vi "Puff_using_Arduino_oneshot.vi"(0 "Puff_duration:Sec":dbl=1.0 format="%.2g") -> ()   [LabVIEW 2015]
uses:
  Controls/Post_Process.ctl
  Controls/Setup.ctl
  Globals/Meas_global.vi
panel:
  out "Puff Time used":dbl=1.0 format="%.2g"
  out "Case Currently On":string="Loop"
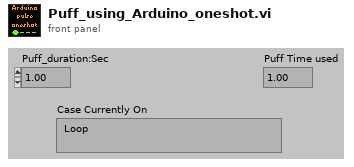
[diagram p1: front panel]
types:
  T1 = typedef "Setup.ctl" = enum16{"Run Program", "Show Setup", "Save Current Setup", "Setup Front Panel"}
  T2 = typedef "Post_Process.ctl" = enum16{"Take New Data", "Post Process Raw Data File"}
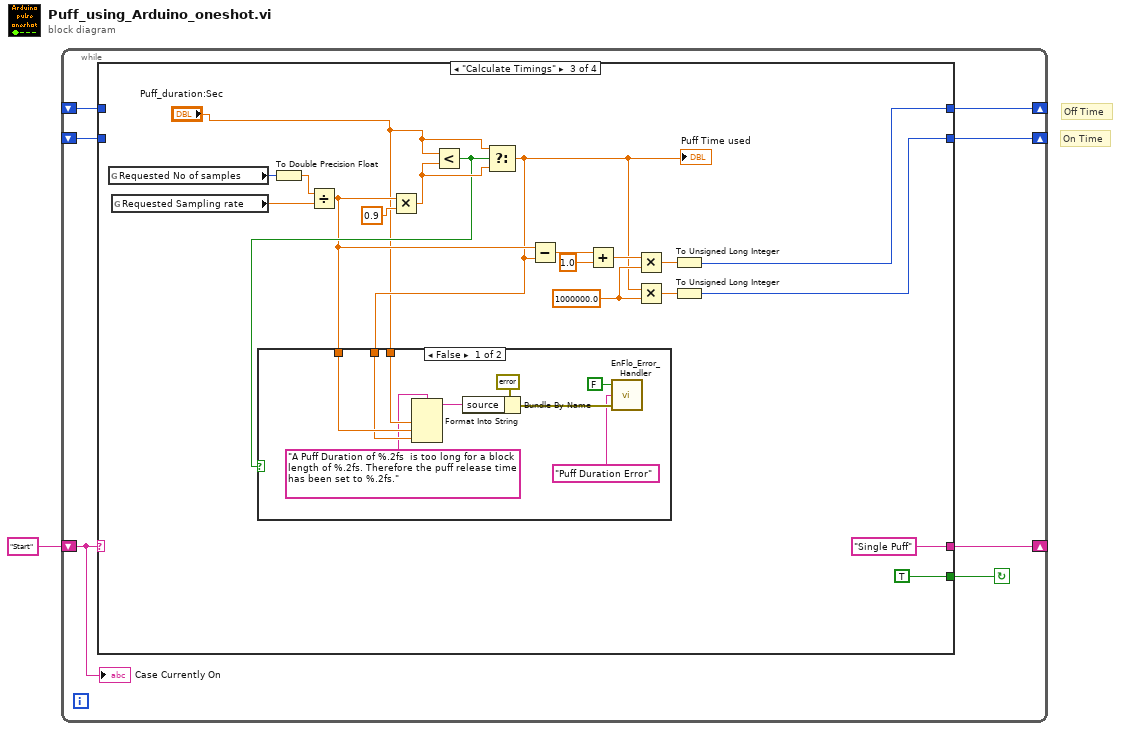
[diagram p0: block diagram]
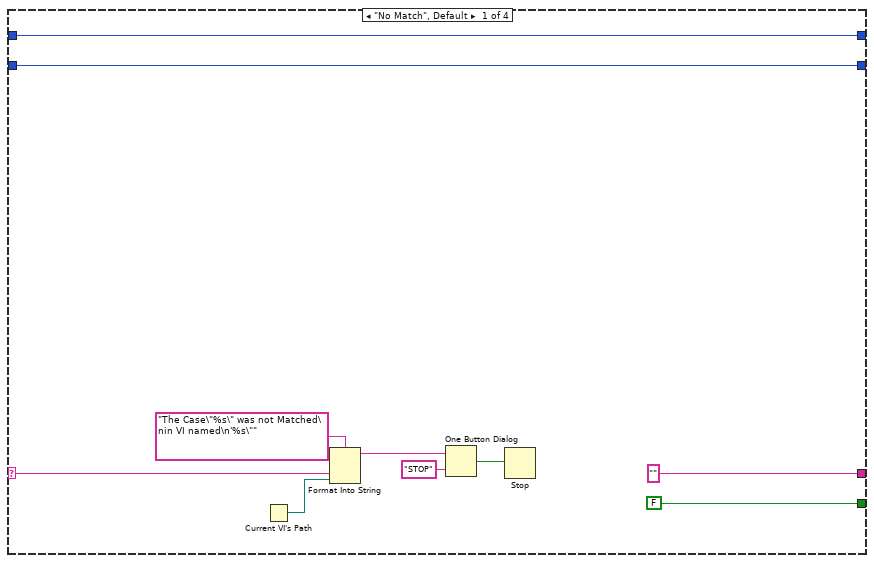
[diagram p2: hidden frame]
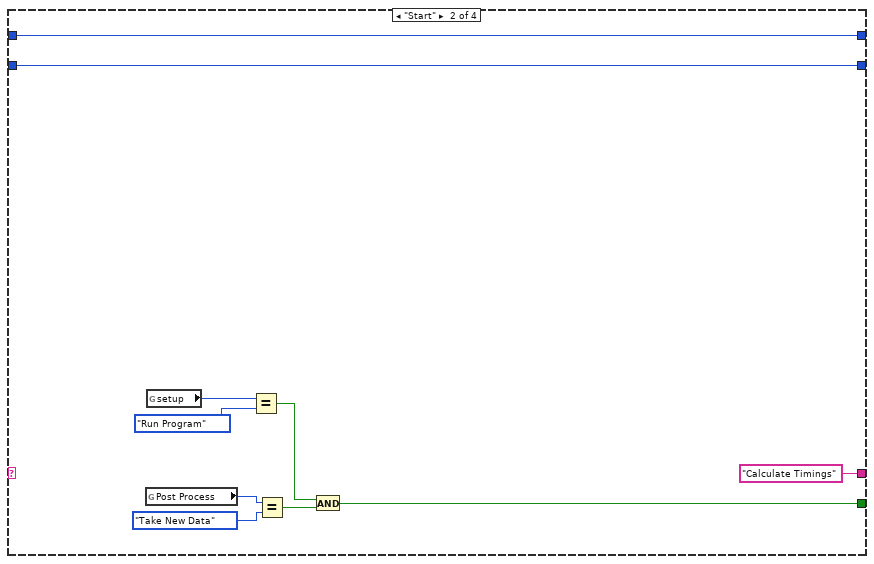
[diagram p3: hidden frame]
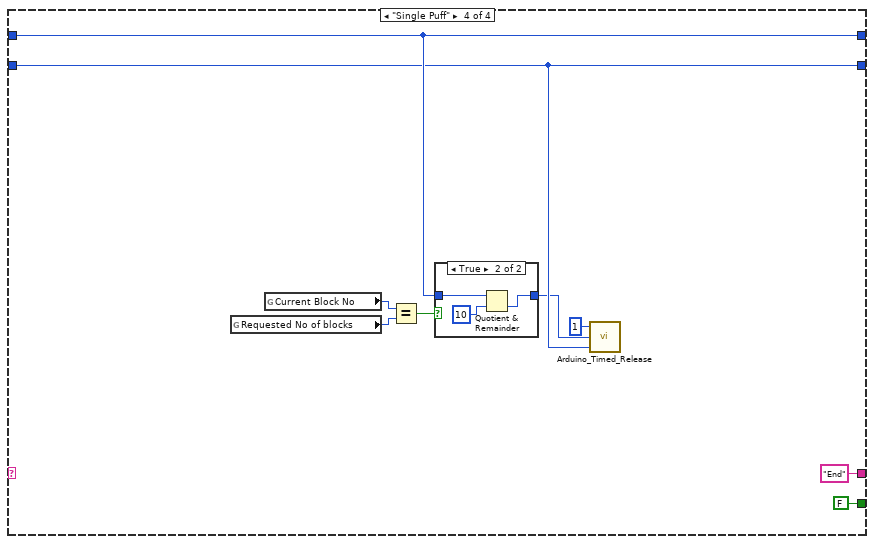
[diagram p5: hidden frame]
diagram:
  # "On Time"
  # "Off Time"
  n1 = while {
    shift-left: "Start" -> [w6]
    shift-right: [w7] -> _
    shift-right: [w5] -> _
    shift-left: _ -> [w4]
    shift-right: [w3] -> _
    shift-left: _ -> [w2]
    stop <- w8 continue-if-true
    n2 = case shown="\"Calculate Timings\"" w6 {
      selector: w6 -> [w9 _ _ _]
      tunnel: [FALSE w21 TRUE ("Command Found") FALSE ("Command Found")] -> w8
      tunnel: ["" "Calculate Timings" "Single Puff" "End"] -> w7
      tunnel: [w11 w20 w32 w65] -> w5
      tunnel: w4 -> [w11 w20 _ w65]
      tunnel: [w10 w19 w31 w64] -> w3
      tunnel: w2 -> [w10 w19 _ w64]
      frame "No Match", Default {
        n3 = Current VI's Path() -> (path=w13:path)
        n4 = Format Into String(format string="The Case\"%s\" was not Matched\nin VI named\n'%s\"" ("Format String"), w9, w13) -> (resulting string=w16:string)  [unwired: 2 in, 1 out]
        n5 = One Button Dialog(message=w16, button name ("OK")="STOP") -> (true=w14:bool)
        n6 = Stop(stop? (T)=w14) -> ()
      }
      frame "Start" {
        n7 = global read "Meas_global.vi" "Post Process"() -> (w23:T2)
        n8 = global read "Meas_global.vi" "setup"() -> (w22:T1)
        n9 = Equal?(x=w22, y=Setup."Run Program") -> (x = y?=w27:bool)
        n10 = Equal?(x=w23, y=Post_Process."Take New Data" ("Post Process")) -> (x = y?=w26:bool)
        n11 = And(x=w27, y=w26) -> (x .and. y?=w21:bool)
      }
      frame "Calculate Timings" {
        w40 = 1000000.0 ("y")
        n12 = global read "Meas_global.vi" "Requested No of samples"() -> (w45:i32)
        n13 = global read "Meas_global.vi" "Requested Sampling rate"() -> (w35:dbl)
        n14 = To Double Precision Float(number=w45) -> (double precision float=w30:dbl)
        n15 = Divide(x=w30, y=w35) -> (x/y=w34:dbl)
        n16 = Multiply(x=w34, y=0.9) -> (x*y=w43:dbl)
        n17 = Less?(x="Puff_duration:Sec", y=w43) -> (x < y?=w36:bool)
        n18 = Select(t="Puff_duration:Sec", s=w36, f=w43) -> (s? t:f=w33:dbl)
        "Puff Time used" <- w33
        n19 = case shown="False" w36 {
          tunnel: "Puff_duration:Sec" -> [w54 _]
          tunnel: w34 -> [w53 _]
          tunnel: w33 -> [w52 _]
          frame False {
            n20 = Format Into String(format string="A Puff Duration of %.2fs  is too long for a block length of %.2fs. Therefore the puff release time has been set to %.2fs.", w54, w53, w52) -> (resulting string=w50:string)  [unwired: 2 in, 1 out]
            n21 = Bundle By Name(cluster=errorcluster {"status"=TRUE, "code"=0, "source"=""} ("error in (no error)"), "source"=w50) -> (w55:errorcluster)
            n22 = call "EnFlo_Error_Handler.vi"("error in (no error)"=w55, "Error Type"="Puff Duration Error", "Dialog Box (T)"=FALSE) -> ()  [unwired: 3 out]
          }
          frame True {
          }
        }
        n23 = Subtract(x=w34, y=w33) -> (x-y=w39:dbl)
        n24 = Add(x=w39, y=1.0) -> (x+y=w37:dbl)
        n25 = Multiply(x=w37, y=w40) -> (x*y=w41:dbl)
        n26 = Multiply(x=w33, y=w40) -> (x*y=w42:dbl)
        n27 = To Unsigned Long Integer(number=w41) -> (unsigned 32bit integer=w32:u32)
        n28 = To Unsigned Long Integer(number=w42) -> (unsigned 32bit integer=w31:u32)
      }
      frame "Single Puff" {
        n29 = global read "Meas_global.vi" "Requested No of blocks"() -> (w59:i32)
        n30 = global read "Meas_global.vi" "Current Block No"() -> (w58:i32)
        n31 = Equal?(x=w58, y=w59) -> (x = y?=w57:bool)
        n32 = case shown="True" w57 {
          tunnel: w65 -> [w66 w69]
          tunnel: [w66 w67] -> w60
          frame False {
          }
          frame True {
            n33 = Quotient & Remainder(x=w69, y=u32 10) -> (floor(x/y)=w67:u32)  [unwired: 1 out]
          }
        }
        n34 = call "Arduino_Timed_Release.vi"("Time to hold source ON (microseconds)"=w64, "Time to hold source OFF (microseconds)"=w60, "Number of cycles"=u16 1) -> ()  [unwired: 2 out]
      }
    }
    "Case Currently On" <- w6
  }
